vi "Select Ring Text Item.vi"(8 "error in (no error)":errorcluster, 10 "Desired Item":string, 11 "Ring":refnum<vi>) -> (0 "error out":errorcluster)   [LabVIEW 2015, in "Utility.lvlib"]
uses:
  Utility.lvlib
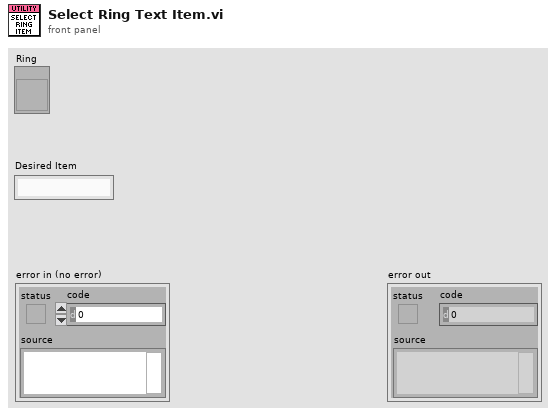
[diagram p1: front panel]
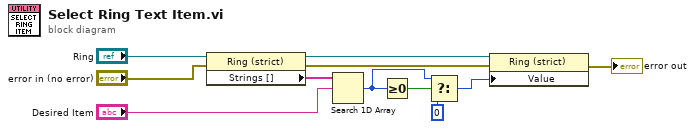
[diagram p0: block diagram]
diagram:
  n1 = property class="Ring (strict)"(reference="Ring", error in="error in (no error)") -> (reference out=w4:refnum<vi>, error out=w2:errorcluster, "Strings []"=w10:string[])
  n2 = Search 1D Array(1D array=w10, element="Desired Item") -> (index of element=w7:i32)  [unwired: 1 in]
  n3 = Greater Or Equal To 0?(x=w7) -> (x >= 0?=w8:bool)
  n4 = Select(t=w7, s=w8, f=0) -> (s? t:f=w6:i32)
  n5 = property class="Ring (strict)"(reference=w4, error in=w2, "Value"=w6) -> (error out=→"error out":errorcluster)  [unwired: 1 out]
